vi "AO Remains.vi"(11 "Array":T1(array[cluster])) -> (0 "String":string, 1 "AO":dbl[](array[numeric]), 2 "Same AO":T1(array[cluster]), 3 "Remains AO":T1(array[cluster]))   [LabVIEW 2022 SP3]
uses:
  RT Controls/AO FGV.ctl
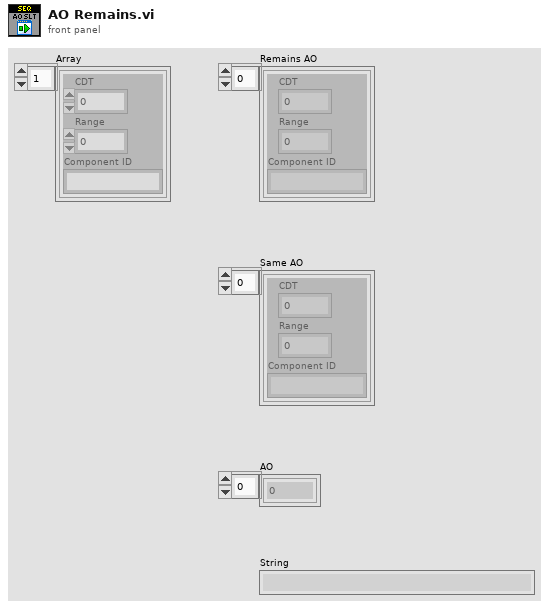
[diagram p1: front panel]
types:
  T1 = cluster{"CDT":dbl, "Range":dbl, "Component ID":string}[]
  T2 = typedef "AO FGV.ctl" = enum16{"Read", "Write", "Start time", "init", "Read Only"}
  T3 = cluster{"CDT":dbl, "Range":dbl, "Component ID":string}
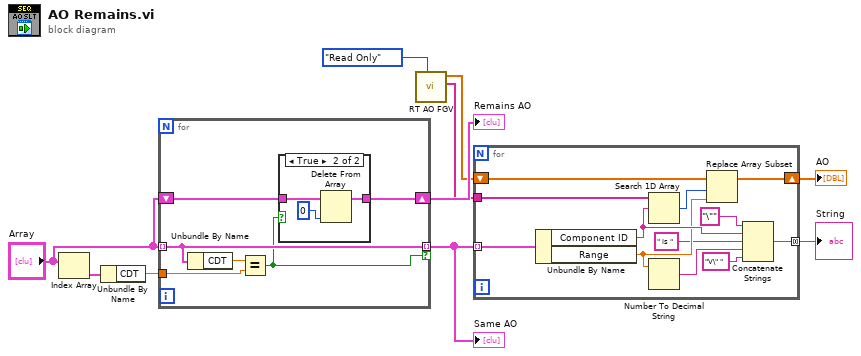
[diagram p0: block diagram]
diagram:
  n1 = Index Array(array="Array") -> (element=w7:T3)  [unwired: 1 in]
  n2 = Unbundle By Name(w7) -> ("CDT"=w9:dbl)
  n3 = for {
    tunnel: "Array" -> [w12] mode=indexing
    shift-right: [w15] -> w10
    shift-left: "Array" -> [w16]
    tunnel: w9 -> [w13]
    tunnel: [w12] -> w6 mode=indexing if=w11
    n4 = Unbundle By Name(w12) -> ("CDT"=w14:dbl)
    n5 = Equal?(x=w14, y=w13) -> (x = y?=w11:bool)
    n6 = case shown="True" w11 {
      tunnel: w16 -> [w17 w20]
      tunnel: [w17 w19] -> w15
      frame False {
      }
      frame True {
        n7 = Delete From Array(array=w20, index=0) -> (array with subset deleted=w19:T1)  [unwired: 1 in, 1 out]
      }
    }
  }
  "Remains AO" <- w10
  "Same AO" <- w6
  n8 = call "RT AO FGV.vi"("Enum"=AO_FGV."Read Only") -> ("AO  Names out"=w3:string[], "AO out"=w2:dbl[])  [unwired: 8 in, 1 out]
  n9 = for {
    tunnel: w6 -> [w32] mode=indexing
    tunnel: w3 -> [w31]
    shift-right: [w28] -> w5
    shift-left: w2 -> [w30]
    tunnel: [w22] -> w1 mode=concatenating
    n10 = Unbundle By Name(w32) -> ("Component ID"=w27:string, "Range"=w26:dbl)
    n11 = Search 1D Array(1D array=w31, element=w27) -> (index of element=w29:i32)  [unwired: 1 in]
    n12 = Number To Decimal String(number=w26) -> (decimal integer string=w24:string)  [unwired: 1 in]
    n13 = Replace Array Subset(array=w30, new element=w26, index=w29) -> (w28:dbl[])
    n14 = Concatenate Strings("\"" ("string"), w27, " is " ("string"), w24, "V\" " ("string")) -> (w22:string)
  }
  "AO" <- w5
  "String" <- w1
